vi "logrecordnumberarray2D.vi"(7 "logsetting":enum16{"error", "info", "debug"}(ring), 8 "error in":errorcluster, 9 "logtype":enum16{"error", "info", "debug"}(ring), 10 "LogPath":path, 11 "Msg":dbl[][](array[numeric])) -> (0 "error out":errorcluster)   [LabVIEW 2011]
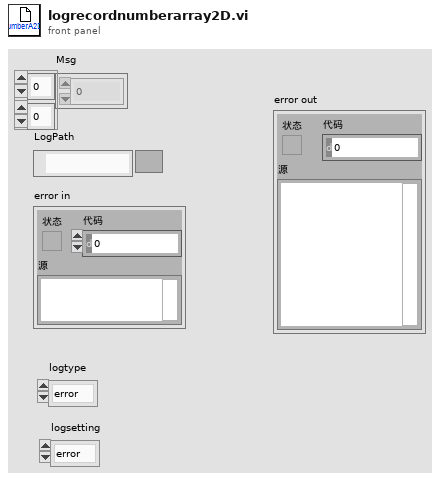
[diagram p1: front panel]
types:
  T1 = enum16{"open", "replace", "create", "open or create", "replace or create", "replace or create with confirmation"}
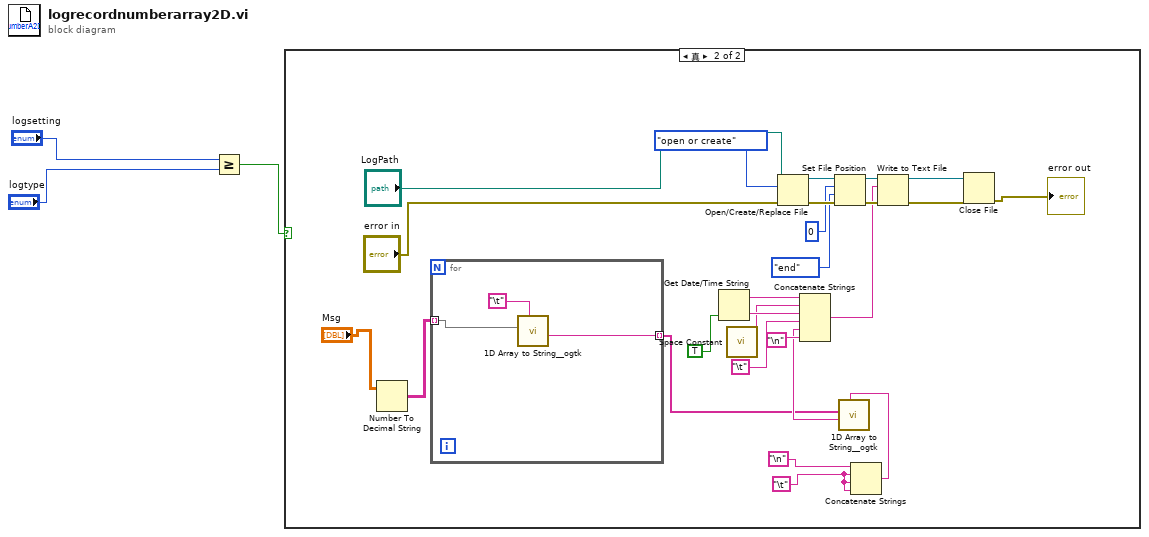
[diagram p0: block diagram]
diagram:
  n1 = Greater Or Equal?(x="logsetting", y="logtype") -> (x >= y?=w1:bool)
  n2 = case shown="真" w1 {
    frame False {
    }
    frame True {
      w8 = "\t"
      n3 = Number To Decimal String(number="Msg") -> (decimal integer string=w4:string[][])  [unwired: 1 in]
      n4 = for {
        tunnel: w4 -> [w32] mode=indexing
        tunnel: [w30] -> w6 mode=indexing
        n5 = call <userlib>:"1D Array to String__ogtk.vi"("delimiter (Tab)"="\t", "Array of Strings"=w32) -> ("delimited string"=w30:string)  [unwired: 9 in]
      }
      n6 = Get Date/Time String(want seconds? (F)=TRUE ("需要秒？(F)")) -> (date string=w16:string, time string=w18:string)  [unwired: 2 in]
      n7 = call <vilib>:"Space Constant.vi"() -> ("String"=w17:string)
      n8 = Open/Create/Replace File(file path (use dialog)="LogPath", error in="error in", operation (0:open)=T1."open or create" ("操作(0:open)")) -> (refnum out=w12:refnum<file>, error out=w22:errorcluster)  [unwired: 3 in, 1 out]
      n9 = Set File Position(offset (in bytes) (0)=i64 0 ("偏移量（字节）（0）"), refnum=w12, from (0:start)=enum16{"start", "end", "current"}."end" ("自（0:起始）"), error in=w22) -> (refnum out=w14:refnum<file>, error out=w23:errorcluster)
      n10 = Concatenate Strings("\n", w8, w8, w8) -> (w9:string)
      n11 = call <userlib>:"1D Array to String__ogtk.vi"("delimiter (Tab)"=w9, "Array of Strings"=w6) -> ("delimited string"=w11:string)  [unwired: 9 in]
      n12 = Concatenate Strings(w16, w17, w18, "\t", w11, "\n") -> (w20:string)
      n13 = Write to Text File(file (use dialog)=w14, text=w20, error in=w23) -> (refnum out=w25:refnum<file>, error out=w26:errorcluster)  [unwired: 1 in, 1 out]
      n14 = Close File(refnum=w25, error in=w26) -> (error out=→"error out":errorcluster)  [unwired: 1 out]
    }
  }
